vi "Query servo for status information.vi"(4 "error in (no error)":errorcluster, 7 "connection in":variant) -> (0 "error out":errorcluster, 1 "Servo variables":T1, 2 "Servo constants":T2={"Name"=enum."AxisX", "Pos position limit [mm]"=0.0, "Neg position limit [mm]"=0.0, "Pos velocity limit"=0.0, "Neg velocity limit"=0.0, "Acceleration limit"=0.0}, 3 "connection out":variant)   [LabVIEW 2021, in "Servo drive module.lvlib"]
uses:
  Servo drive module.lvlib
  ctl/Servo constants.ctl
  ctl/Servo variables.ctl
  ctl/Axis names.ctl
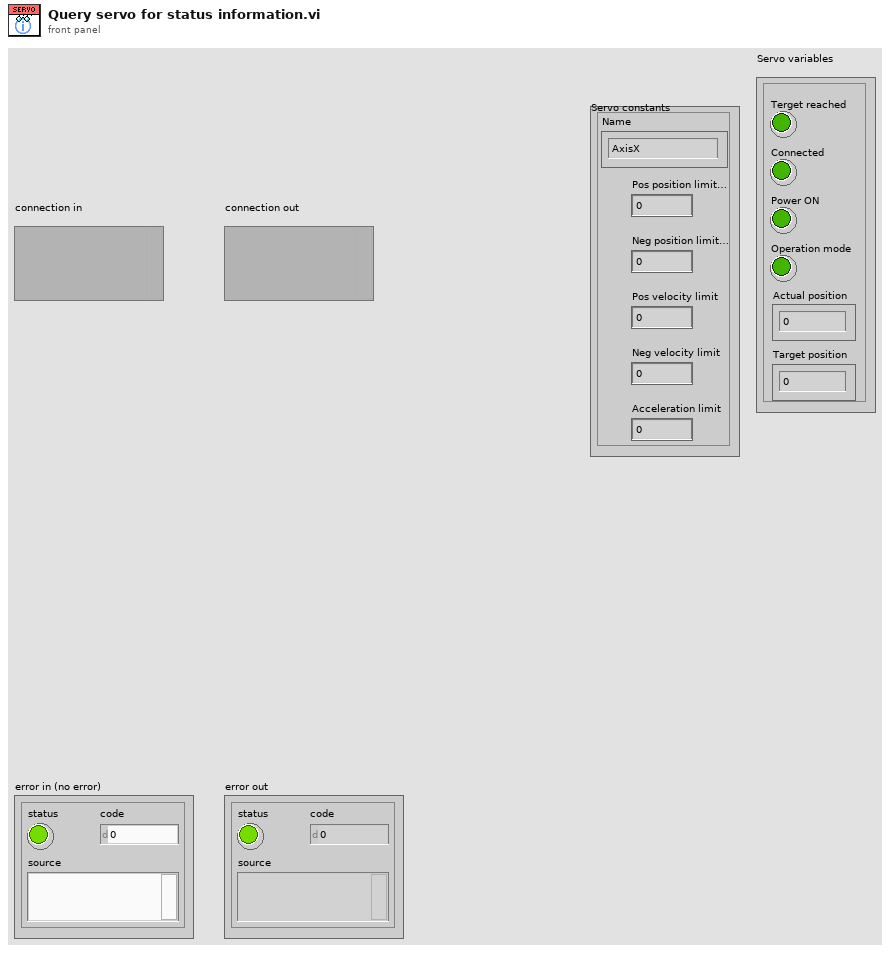
[diagram p1: front panel]
types:
  T1 = typedef "Servo drive module.lvlib/Servo variables.ctl" = cluster{"Terget reached":bool, "Connected":bool, "Power ON":bool, "Operation mode":bool, "Actual position":dbl, "Target position":dbl}
  T2 = typedef "Servo drive module.lvlib/Servo constants.ctl" = cluster{"Name":T3, "Pos position limit [mm]":dbl, "Neg position limit [mm]":dbl, "Pos velocity limit":dbl, "Neg velocity limit":dbl, "Acceleration limit":dbl}
  T3 = typedef "Servo drive module.lvlib/Axis names.ctl" = enum16{"Unknown", "AxisX", "AxisY", "AxisZ_left", "AxisZ_middle", "AxisZ_right"}
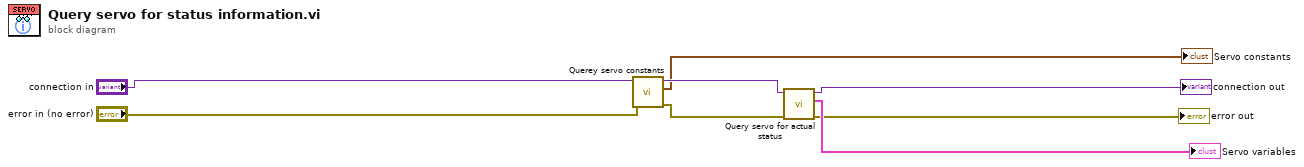
[diagram p0: block diagram]
diagram:
  n1 = call "Querey servo constants.vi"("error in (no error)"="error in (no error)", "connection in"="connection in") -> ("error out"=w7:errorcluster, "Servo constants"=→"Servo constants":T2, "connection out"=w2:variant)  [unwired: 7 in]
  n2 = call "Query servo for actual status.vi"("error in (no error)"=w7, "connection in"=w2) -> ("error out"=→"error out":errorcluster, "Servo variables"=→"Servo variables":T1, "connection out"=→"connection out":variant)  [unwired: 7 in]
